vi "FileInput.vi"() -> ()   [LabVIEW 2019]
panel:
  out "Input File":string
  out "Output Array":dbl[][](array[numeric])
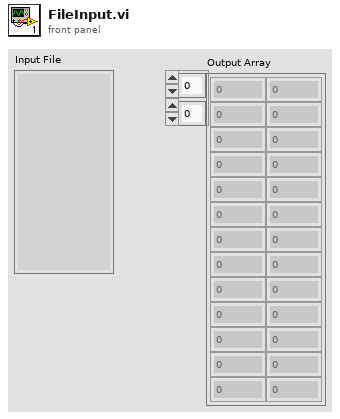
[diagram p1: front panel]
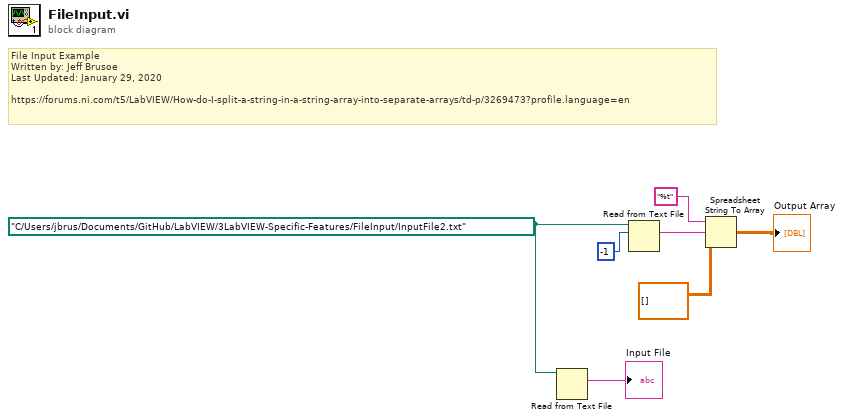
[diagram p0: block diagram]
diagram:
  w3 = path "C:/Users/jbrus/Documents/GitHub/LabVIEW/3LabVIEW-Specific-Features/FileInput/InputFile2.txt"
  # "File Input Example\nWritten by: Jeff Brusoe\nLast Updated: January 29, 2020\n\nhttps://forums.ni.com/t5/LabVIEW/How-do-I-split-a-string-in-a-string-array-into-separate-arrays/td-p/3269473?profile.language=en"
  n1 = Read from Text File(file (use dialog)=w3) -> (text=→"Input File":string)  [unwired: 3 in, 3 out]
  n2 = Read from Text File(file (use dialog)=w3, count=-1) -> (text=w7:string)  [unwired: 2 in, 3 out]
  n3 = Spreadsheet String To Array(format string="%t", spreadsheet string=w7, array type (2D Dbl)=dbl[][] []) -> (array=→"Output Array":dbl[][])  [unwired: 1 in]
